vi "Control Panel 9620 (no objects).vi"() -> ()   [LabVIEW 2023]
uses:
  Global/GPIB Numbers.vi
  <vilib>/Analysis/NI_AALBase.lvlib
panel:
  in  "index":i32
  out "standard\ndeviation":dbl format="%0.2f"
  in  "X":dbl[](array[numeric]) format="%0.2f"
  in  "Announcement":bool
  in  "Announce":dbl
  out "Current \nheater output":dbl format="%_4g"
  in  "Toggle control mode":bool
  out "updating values":bool
  out "error out":errorcluster
  in  "error in":errorcluster
  in  "Change set \ntemperature":dbl min=0.0 max=300.0
  out "Current set\ntemperature":dbl
  out "Current \ntemperature":dbl
  in  "stop":bool
  # "%"
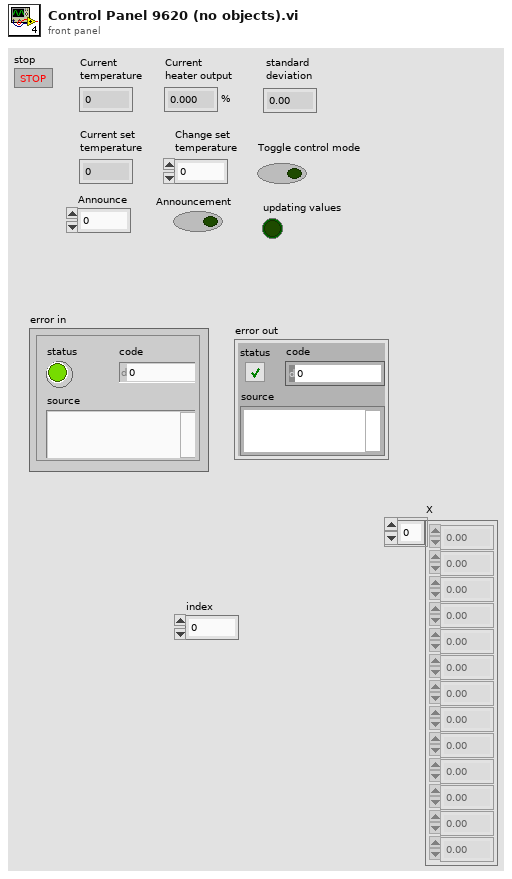
[diagram p1: front panel]
types:
  T1 = typedef "GPIB Type Def.ctl" = cluster{"Name":string, "bus":dbl, "GPIB":dbl, "GPIB as string":string, "byte":i32, "VISA Resource Name":refnum<visa-resource-name>}
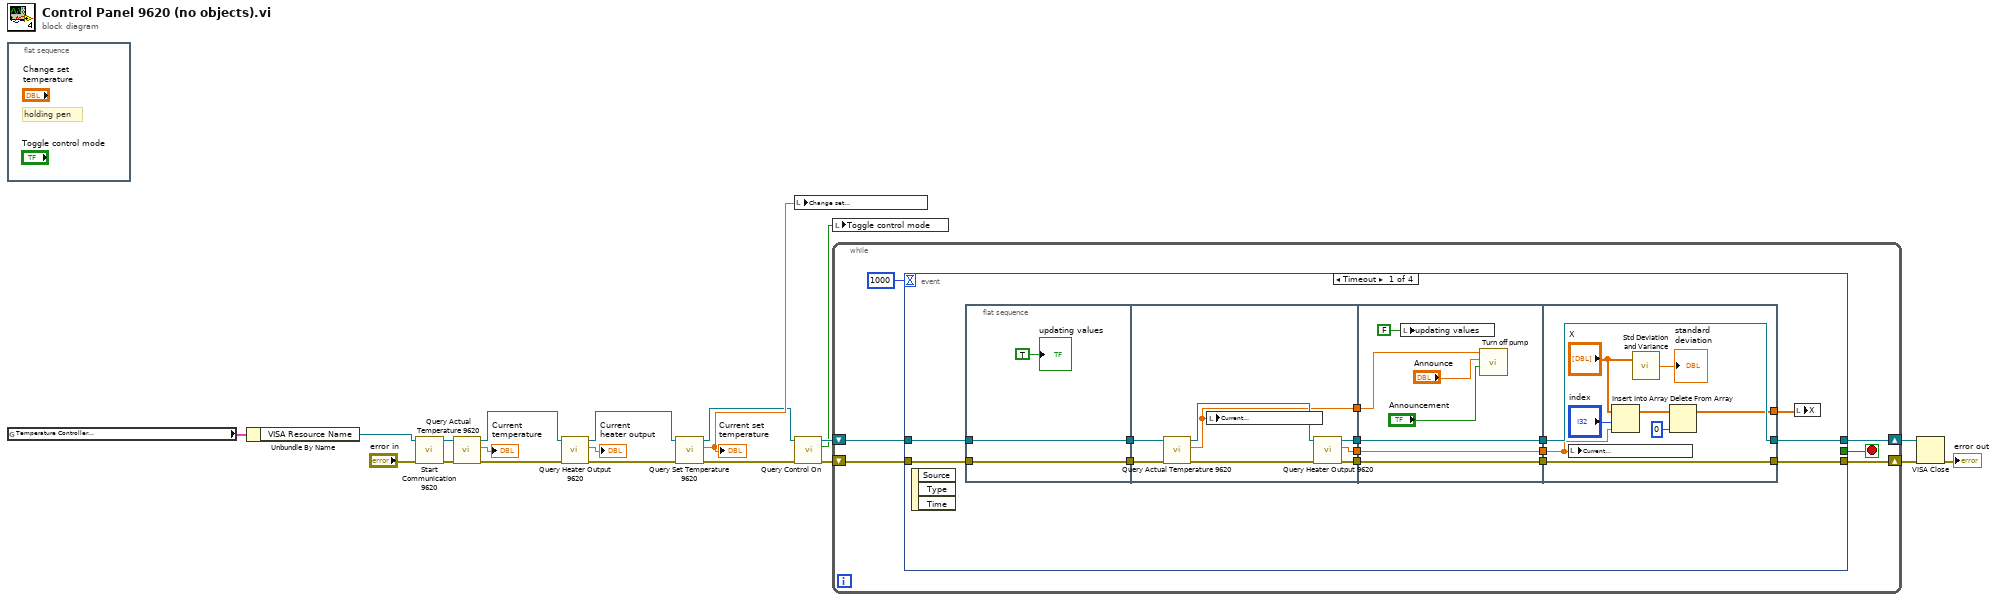
[diagram p0: block diagram]
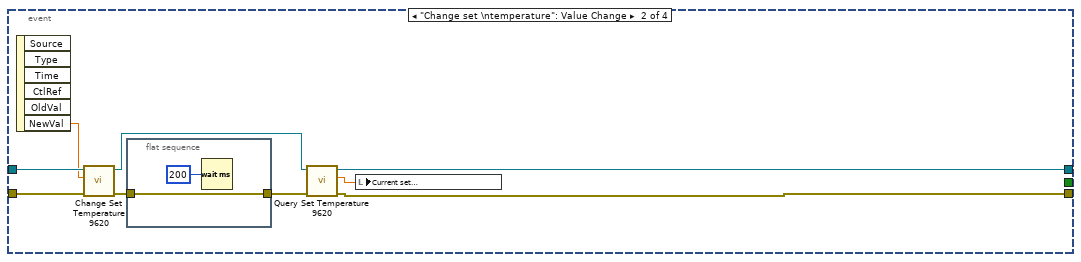
[diagram p2: hidden frame]
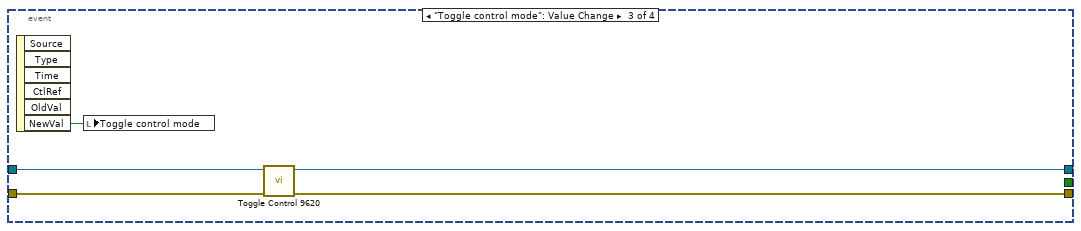
[diagram p3: hidden frame]
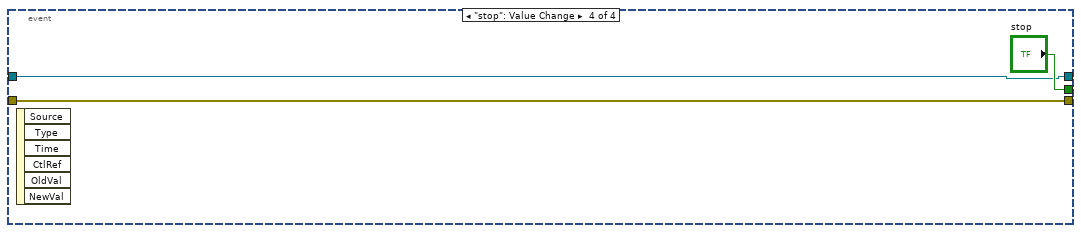
[diagram p4: hidden frame]
diagram:
  n1 = flat-sequence {
    frame #0 {
      # "holding pen"
    }
  }
  n2 = global read "GPIB Numbers.vi" "Temperature Controller\nScientific Instruments"() -> (w20:T1)
  n3 = Unbundle By Name(w20) -> ("VISA Resource Name"=w2:refnum<visa-resource-name>)
  n4 = call "Start Communication 9620.vi"("error in"="error in", "VISA resource name"=w2) -> ("error out"=w3:errorcluster, "VISA out"=w1:refnum<visa-resource-name>)  [unwired: 8 in]
  n5 = call "Query Actual Temperature 9620.vi"("error in (no error)"=w3, "VISA resource name"=w1) -> ("error out"=w6:errorcluster, "Current actual temperature"=→"Current \ntemperature":dbl, "VISA resource name out"=w8:refnum<visa-resource-name>)  [unwired: 7 in]
  n6 = call "Query Heater Output 9620.vi"("error in (no error)"=w6, "VISA resource name"=w8) -> ("error out"=w5:errorcluster, "Current heater output"=→"Current \nheater output":dbl, "VISA resource name out"=w7:refnum<visa-resource-name>)  [unwired: 7 in]
  n7 = call "Query Set Temperature 9620.vi"("error in (no error)"=w5, "VISA resource name"=w7) -> ("error out"=w12:errorcluster, "Set temperature"=w18:dbl, "VISA resource name out"=w14:refnum<visa-resource-name>)  [unwired: 7 in]
  "Current set\ntemperature" <- w18
  n8 = local write "Change set \ntemperature"(w18) -> ()
  n9 = call "Query Control On.vi"("error in (no error)"=w12, "VISA resource name"=w14) -> ("error out"=w11:errorcluster, "Control on?"=w10:bool, "VISA resource name out"=w13:refnum<visa-resource-name>)  [unwired: 7 in]
  n10 = local write "Toggle control mode"(w10) -> ()
  n11 = while {
    shift-right: [w24] -> w16
    shift-left: w11 -> [w25]
    shift-right: [w22] -> w17
    shift-left: w13 -> [w23]
    stop <- w26 stop-if-true
    n12 = event shown="[0] Timeout" {
      selector: _ -> [_ _ _ _]
      dyn-events: _ -> [_ _ _ _]
      timeout: 1000 -> [_ _ _ _]
      tunnel: [_ _ _ "stop"] -> w26
      tunnel: w25 -> [w38 w75 w82 w85]
      tunnel: [w37 w71 w80 w85] -> w24
      tunnel: w23 -> [w40 w76 w83 w84]
      tunnel: [w39 w70 w81 w84] -> w22
      event Timeout {
        n13 = event-data() -> ()  [unwired: 1 in, 3 out]
        n14 = flat-sequence {
          tunnel: w38 -> [w42]
          tunnel: w40 -> [w43]
          tunnel: [w43] -> w36
          tunnel: [w42] -> w35
          tunnel: w36 -> [w51]
          tunnel: w35 -> [w50]
          tunnel: [w48] -> w34
          tunnel: [w46] -> w33
          tunnel: [w45] -> w32
          tunnel: [w44] -> w28
          tunnel: w34 -> [w58]
          tunnel: w33 -> [w57]
          tunnel: w32 -> [w55]
          tunnel: [w58] -> w31
          tunnel: [w57] -> w30
          tunnel: [w52] -> w29
          tunnel: w28 -> [w52]
          tunnel: [w66] -> w37
          tunnel: [w67] -> w39
          tunnel: w31 -> [w67]
          tunnel: w30 -> [w66]
          tunnel: w29 -> [w65]
          tunnel: [w59] -> w27
          frame #0 {
            "updating values" <- TRUE ("updating value")
          }
          frame #1 {
            n15 = call "Query Actual Temperature 9620.vi"("error in (no error)"=w50, "VISA resource name"=w51) -> ("error out"=w47:errorcluster, "Current actual temperature"=w45:dbl, "VISA resource name out"=w49:refnum<visa-resource-name>)  [unwired: 7 in]
            n16 = local write "Current \ntemperature"(w45) -> ()
            n17 = call "Query Heater Output 9620.vi"("error in (no error)"=w47, "VISA resource name"=w49) -> ("error out"=w46:errorcluster, "Current heater output"=w44:dbl, "VISA resource name out"=w48:refnum<visa-resource-name>)  [unwired: 7 in]
          }
          frame #2 {
            n18 = local write "updating values"(FALSE ("updating value")) -> ()
            n19 = call "Turn off pump.vi"("Boolean"="Announcement", "Announce"="Announce", "Numeric"=w55) -> ()  [unwired: 9 in]
          }
          frame #3 {
            n20 = local write "Current \nheater output"(w65) -> ()
            n21 = Insert Into Array(array="X", index="index", new element=w65) -> (w60:dbl[])
            n22 = call <vilib>:"Std Deviation and Variance.vi"("X"="X") -> ("standard deviation"=→"standard\ndeviation":dbl)  [unwired: 1 in, 2 out]
            n23 = Delete From Array(array=w60, index=0) -> (array with subset deleted=w59:dbl[])  [unwired: 1 in, 1 out]
          }
        }
        n24 = local write "X"(w27) -> ()
      }
      event "Change set \ntemperature": Value Change {
        n25 = event-data() -> ("NewVal"=w69:dbl)  [unwired: 1 in, 5 out]
        n26 = call "Change Set Temperature 9620.vi"("error in (no error)"=w75, "Temperture Setpoint"=w69, "VISA resource name"=w76) -> ("error out"=w74:errorcluster, "VISA resource name out"=w73:refnum<visa-resource-name>)  [unwired: 7 in]
        n27 = flat-sequence {
          tunnel: [w77] -> w72
          tunnel: w74 -> [w77]
          frame #0 {
            n28 = Wait (ms)(milliseconds to wait=u32 200) -> ()  [unwired: 1 out]
          }
        }
        n29 = call "Query Set Temperature 9620.vi"("error in (no error)"=w72, "VISA resource name"=w73) -> ("error out"=w71:errorcluster, "Set temperature"=w68:dbl, "VISA resource name out"=w70:refnum<visa-resource-name>)  [unwired: 7 in]
        n30 = local write "Current set\ntemperature"(w68) -> ()
      }
      event "Toggle control mode": Value Change {
        n31 = event-data() -> ("NewVal"=w79:bool)  [unwired: 1 in, 5 out]
        n32 = local write "Toggle control mode"(w79) -> ()
        n33 = call "Toggle Control 9620.vi"("error in (no error)"=w82, "VISA resource name"=w83) -> ("error out"=w80:errorcluster, "VISA resource name out"=w81:refnum<visa-resource-name>)  [unwired: 8 in]
      }
      event "stop": Value Change {
        n34 = event-data() -> ()  [unwired: 1 in, 6 out]
      }
    }
  }
  n35 = VISA Close(VISA resource name=w17, error in (no error)=w16) -> (error out=→"error out":errorcluster)
